vi "Get Empty Cluster.vi"(8 "error in (no error)":errorcluster) -> (0 "error out":errorcluster, 3 "Cluster out":variant)   [LabVIEW 2017, in "Cluster Manipulation API.lvlib"]
uses:
  Cluster Manipulation API.lvlib
  <vilib>/Utility/Data Type/NI_Data Type.lvlib
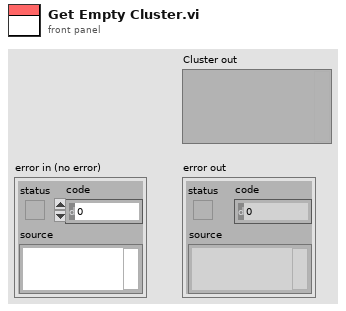
[diagram p1: front panel]
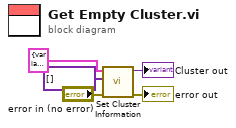
[diagram p0: block diagram]
diagram:
  n1 = call <vilib>:"Set Cluster Information.vi"("error in (no error)"="error in (no error)", "Cluster Elements"=variant[] [], "Variant in"=cluster{variant} {variant}) -> ("error out"=→"error out":errorcluster, "Variant out"=→"Cluster out":variant)  [unwired: 7 in]
